vi "Slice Peak Window.vi"(1 "Padding":u32=3, 2 "Peak Index":dbl, 3 "Target Baseline (%)":dbl, 4 "Intensity Data":dbl[](array[numeric])) -> (0 "Peak Window (X,Y)":cluster{"Indices":u32[], "Sliced Data":dbl[]})   [LabVIEW 2012]
panel:
  out "center -> left":dbl[](graph)
  out "center -> right":dbl[](graph)
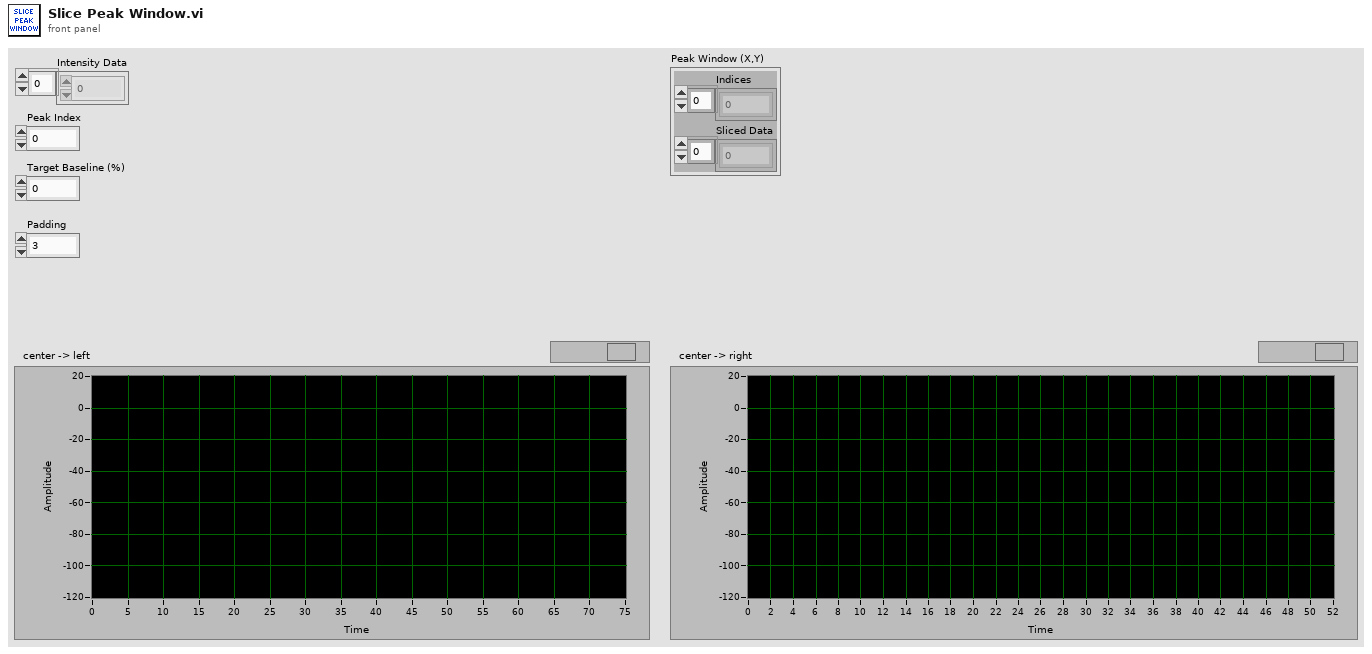
[diagram p1: front panel]
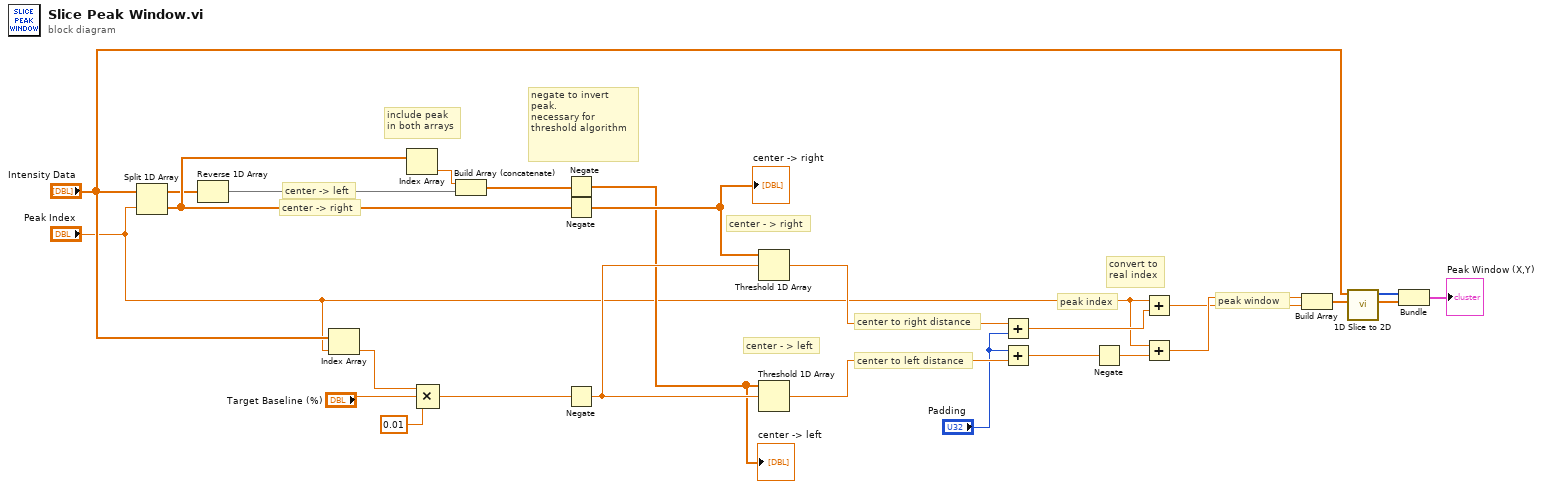
[diagram p0: block diagram]
diagram:
  # "peak index"
  # "peak window"
  # "center to right distance"
  # "center to left distance"
  # "center -> right"
  # "center -> left"
  # "include peak\nin both arrays"
  # "negate to invert peak.\nnecessary for threshold algorithm"
  # "center - > left"
  # "center - > right"
  # "convert to\nreal index"
  n1 = Split 1D Array(array="Intensity Data", index="Peak Index") -> (first subarray=w17:dbl[], second subarray=w21:dbl[])
  n2 = Reverse 1D Array(array=w17) -> (reversed array=w16:dbl[])
  n3 = Index Array(array="Intensity Data", index="Peak Index") -> (element=w4:dbl)
  n4 = Index Array(array=w21) -> (element=w20:dbl)  [unwired: 1 in]
  n5 = Compound Arithmetic op=MULTIPLY(w4, "Target Baseline (%)", 0.01 ("value")) -> (w1:dbl)
  n6 = Build Array (concatenate)(w20, w16) -> (w19:dbl[])
  n7 = Negate(x=w19) -> (-x=w18:dbl[])
  "center -> left" <- w18
  n8 = Negate(x=w21) -> (-x=w23:dbl[])
  "center -> right" <- w23
  n9 = Negate(x=w1) -> (-x=w22:dbl)
  n10 = Threshold 1D Array(2:w22, 3:w23) -> (0:w15:dbl)  [unwired: 1 in]
  n11 = Threshold 1D Array(2:w22, 3:w18) -> (0:w14:dbl)  [unwired: 1 in]
  n12 = Add(x=w15, y="Padding") -> (x+y=w24:dbl)
  n13 = Add(x="Padding", y=w14) -> (x+y=w25:dbl)
  n14 = Negate(x=w25) -> (-x=w26:dbl)
  n15 = Add(x="Peak Index", y=w24) -> (x+y=w10:dbl)
  n16 = Add(x="Peak Index", y=w26) -> (x+y=w12:dbl)
  n17 = Build Array(w12, w10) -> (w11:dbl[])
  n18 = call "1D Slice to 2D.vi"("Fit Range"=w11, "Data In"="Intensity Data") -> ("Sliced Data"=w8:dbl[], "Indices"=w9:u32[])  [unwired: 7 in, 1 out]
  n19 = Bundle("Indices"=w9, "Sliced Data"=w8) -> (→"Peak Window (X,Y)":cluster{"Indices":u32[], "Sliced Data":dbl[]})  [unwired: 1 in]
